vi "LV2_User_Event_Operations.vi"(0 "Event Data":dbl, 11 "Error In":errorcluster, 13 "Operation":T1) -> (4 "Event Data":refnum<user-event>, 15 "Error Out":errorcluster)   [LabVIEW 2020]
doc: "User Event LV 2 Global Variable"
uses:
  Typedef/LV2_User_Event.ctl
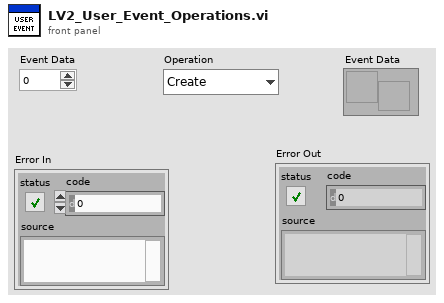
[diagram p1: front panel]
types:
  T1 = typedef "LV2_User_Event.ctl" = enum16{"Create", "Generate", "Read", "Destroy"}
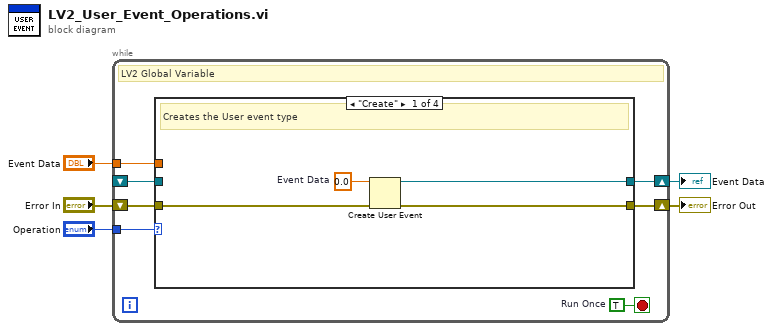
[diagram p0: block diagram]
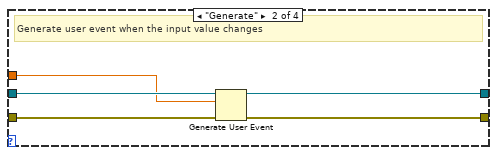
[diagram p2: hidden frame]
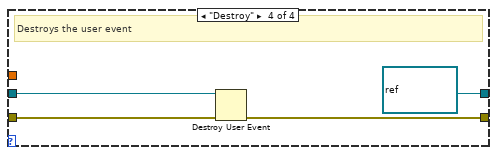
[diagram p4: hidden frame]
diagram:
  n1 = while {
    tunnel: "Operation" -> [w11]
    shift-right: [w7] -> w2
    shift-left: _ -> [w8]
    shift-right: [w10] -> w3
    shift-left: "Error In" -> [w9]
    tunnel: "Event Data" -> [w6]
    stop <- w12 stop-if-true
    w12 = TRUE  # Run Once
    # "LV2 Global Variable"
    n2 = case shown="\"Create\"" w11 {
      tunnel: [w16 w20 w23 w26] -> w10
      tunnel: w9 -> [w15 w21 w23 w27]
      tunnel: w8 -> [_ w19 w22 w25]
      tunnel: [w14 w18 w22 refnum<user-event> refnum ("Event Data")] -> w7
      tunnel: w6 -> [_ w17 _ _]
      frame "Create" {
        w13 = 0.0  # Event Data
        # "Creates the User event type"
        n3 = Create User Event(user event datatype=w13, error in=w15) -> (user event=w14:refnum<user-event>, error out=w16:errorcluster)
      }
      frame "Generate" {
        # "Generate user event when the input value changes"
        n4 = Generate User Event(user event=w19, event data cluster=w17, error in=w21) -> (user event out=w18:refnum<user-event>, error out=w20:errorcluster)  [unwired: 1 in]
      }
      frame "Read" {
        # "Reads the Generated reference"
      }
      frame "Destroy" {
        # "Destroys the user event"
        n5 = Destroy User Event(user event=w25, error in=w27) -> (error out=w26:errorcluster)
      }
    }
  }
  "Error Out" <- w3
  "Event Data" <- w2
